vi "Lab Panel V5.22.vi"() -> ()   [LabVIEW 2013] (continued)
                    n2880 = Concatenate Strings("]", "\r") -> (w5216:string)
                    n2881 = Concatenate Strings(w5211, w5236, w5216) -> (w5226:string)
                    n2882 = Concatenate Strings(w5213, w5238, w5216) -> (w5228:string)
                    n2883 = Concatenate Strings(w5212, w5237, w5216) -> (w5227:string)
                    n2884 = Concatenate Strings(w5208, w5233, w5216) -> (w5223:string)
                    n2885 = Concatenate Strings(w5209, w5232, w5216) -> (w5224:string)
                    n2886 = Concatenate Strings(w5207, w5234, w5216) -> (w5222:string)
                    n2887 = Concatenate Strings(w5206, w5235, w5216) -> (w5221:string)
                    n2888 = Concatenate Strings(w5210, w5231, w5216) -> (w5225:string)
                    n2889 = Concatenate Strings(w5214, w5239, w5216) -> (w5229:string)
                    n2890 = Concatenate Strings(w5215, w5240, w5216) -> (w5230:string)
                    n2891 = Concatenate Strings(w5230, w5229, w5228, w5227, w5226, w5221, w5222, w5223, w5224, w5225) -> (w5199:string)
                    n2892 = Concatenate Strings("[PANEL/", "DESC/", "CYCLES/", "MINS/", "STATUS]", "\r", w5199) -> (w5198:string)
                    "MAIL REPORT" <- w5198
                    n2893 = global write "Global display 3.vi" "log all"(w5198) -> ()
                  }
                  frame #2 {
                    w5329 = "END"
                    n2894 = local read "mail control"() -> (w5330:string)
                    n2895 = case shown="False" w5325 {
                      tunnel: w5330 -> [w5354 _]
                      tunnel: w5329 -> [w5353 _]
                      tunnel: [w5352 FALSE] -> w5315
                      frame False {
                        n2896 = Equal?(x=w5354, y=w5353) -> (x = y?=w5352:bool)
                      }
                      frame True {
                      }
                    }
                    n2897 = case shown="False" w5331 {
                      tunnel: w5330 -> [w5370 _]
                      tunnel: w5329 -> [w5369 _]
                      tunnel: [w5368 FALSE] -> w5319
                      frame False {
                        n2898 = Equal?(x=w5370, y=w5369) -> (x = y?=w5368:bool)
                      }
                      frame True {
                      }
                    }
                    n2899 = case shown="False" w5328 {
                      tunnel: w5330 -> [w5366 _]
                      tunnel: w5329 -> [w5365 _]
                      tunnel: [w5364 FALSE] -> w5318
                      frame False {
                        n2900 = Equal?(x=w5366, y=w5365) -> (x = y?=w5364:bool)
                      }
                      frame True {
                      }
                    }
                    n2901 = case shown="False" w5326 {
                      tunnel: w5330 -> [w5358 _]
                      tunnel: w5329 -> [w5357 _]
                      tunnel: [w5356 FALSE] -> w5316
                      frame False {
                        n2902 = Equal?(x=w5358, y=w5357) -> (x = y?=w5356:bool)
                      }
                      frame True {
                      }
                    }
                    n2903 = case shown="False" w5327 {
                      tunnel: w5330 -> [w5362 _]
                      tunnel: w5329 -> [w5361 _]
                      tunnel: [w5360 FALSE] -> w5317
                      frame False {
                        n2904 = Equal?(x=w5362, y=w5361) -> (x = y?=w5360:bool)
                      }
                      frame True {
                      }
                    }
                    n2905 = Or(x=w5317, y=w5316) -> (x .or. y?=w5308:bool)
                    n2906 = Or(x=w5319, y=w5318) -> (x .or. y?=w5309:bool)
                    n2907 = Or(x=w5309, y=w5308) -> (x .or. y?=w5304:bool)
                    n2908 = case shown="False" w5321 {
                      tunnel: w5330 -> [w5338 _]
                      tunnel: w5329 -> [w5337 _]
                      tunnel: [w5336 FALSE] -> w5310
                      frame False {
                        n2909 = Equal?(x=w5338, y=w5337) -> (x = y?=w5336:bool)
                      }
                      frame True {
                      }
                    }
                    n2910 = case shown="False" w5320 {
                      tunnel: w5330 -> [w5334 _]
                      tunnel: w5329 -> [w5333 _]
                      tunnel: [w5332 FALSE] -> w5314
                      frame False {
                        n2911 = Equal?(x=w5334, y=w5333) -> (x = y?=w5332:bool)
                      }
                      frame True {
                      }
                    }
                    n2912 = case shown="False" w5322 {
                      tunnel: w5330 -> [w5342 _]
                      tunnel: w5329 -> [w5341 _]
                      tunnel: [w5340 FALSE] -> w5311
                      frame False {
                        n2913 = Equal?(x=w5342, y=w5341) -> (x = y?=w5340:bool)
                      }
                      frame True {
                      }
                    }
                    n2914 = case shown="False" w5324 {
                      tunnel: w5330 -> [w5350 _]
                      tunnel: w5329 -> [w5349 _]
                      tunnel: [w5348 FALSE] -> w5313
                      frame False {
                        n2915 = Equal?(x=w5350, y=w5349) -> (x = y?=w5348:bool)
                      }
                      frame True {
                      }
                    }
                    n2916 = case shown="False" w5323 {
                      tunnel: w5330 -> [w5346 _]
                      tunnel: w5329 -> [w5345 _]
                      tunnel: [w5344 FALSE] -> w5312
                      frame False {
                        n2917 = Equal?(x=w5346, y=w5345) -> (x = y?=w5344:bool)
                      }
                      frame True {
                      }
                    }
                    n2918 = Or(x=w5313, y=w5312) -> (x .or. y?=w5307:bool)
                    n2919 = Or(x=w5311, y=w5310) -> (x .or. y?=w5306:bool)
                    n2920 = Or(x=w5314, y=w5315) -> (x .or. y?=w5302:bool)
                    n2921 = Or(x=w5307, y=w5306) -> (x .or. y?=w5305:bool)
                    n2922 = Or(x=w5304, y=w5305) -> (x .or. y?=w5303:bool)
                    n2923 = Or(x=w5303, y=w5302) -> (x .or. y?=w5301:bool)
                  }
                  frame #3 {
                    n2924 = local read "on loops"() -> (w5384:dbl)
                    n2925 = local read "jig cycle"() -> (w5381:dbl)
                    n2926 = local read "Send Mail Now"() -> (w5375:bool)
                    n2927 = Add(x=w5384, y=3.0) -> (x+y=w5382:dbl)
                    n2928 = Equal?(x=w5381, y=w5382) -> (x = y?=w5376:bool)
                    n2929 = And(x=w5376, y=w5375) -> (x .and. y?=w5374:bool)
                    n2930 = And(x=w5380, y=w5376) -> (x .and. y?=w5379:bool)
                    n2931 = And(x=w5379, y=w5378) -> (x .and. y?=w5377:bool)
                    n2932 = Or(x=w5377, y=w5374) -> (x .or. y?=w5373:bool)
                    n2933 = case shown="True" w5373 {
                      tunnel: w5389 -> [_ w5395]
                      tunnel: w5388 -> [_ w5394]
                      tunnel: "Lab Panel Test Status" -> [_ w5393]
                      tunnel: w5386 -> [_ w5392]
                      tunnel: w5385 -> [_ w5391]
                      tunnel: w5372 -> [_ w5390]
                      frame False {
                      }
                      frame True {
                        n2934 = stacked-sequence {
                          tunnel: w5395 -> [w5403 _]
                          tunnel: w5394 -> [w5402 _]
                          tunnel: w5393 -> [w5401 _]
                          tunnel: w5392 -> [w5400 _]
                          tunnel: w5391 -> [w5399 _]
                          tunnel: w5390 -> [w5398 _]
                          frame #0 {
                            n2935 = call "sub vi - send mail v5.vi"("TO:"=w5403, "subject"=w5401, "from"=w5399, "out going server"=w5400, "message"=w5402) -> ("error out"=w5397:errorcluster)  [unwired: 10 in]
                            n2936 = Bundle(cluster=w5398, "mail error"=w5397) -> (w5396:T7)  [unwired: 6 in]
                            n2937 = local write "MAIL SETTINGS"(w5396) -> ()
                          }
                          frame #1 {
                            n2938 = local write "mail control"("") -> ()
                            n2939 = local write "Send Mail Now"(FALSE) -> ()
                          }
                        }
                      }
                    }
                  }
                }
              }
            }
          }
          frame #18 {
            # "save jig cycle values once all run switches are off"
            n2940 = stacked-sequence {
              tunnel: w5415 -> [_ w5444]
              tunnel: w5414 -> [_ w5443]
              tunnel: w5413 -> [_ w5442]
              tunnel: w5412 -> [_ w5441]
              tunnel: w5411 -> [_ w5440]
              tunnel: w5410 -> [_ w5439]
              tunnel: w5409 -> [_ w5438]
              tunnel: w5408 -> [_ w5437]
              tunnel: w5407 -> [_ w5436]
              tunnel: w5406 -> [_ w5435]
              frame #0 {
              }
              frame #1 {
                n2941 = Not(x=w5435) -> (.not. x?=w5418:bool)
                n2942 = Not(x=w5443) -> (.not. x?=w5433:bool)
                n2943 = Not(x=w5440) -> (.not. x?=w5428:bool)
                n2944 = Not(x=w5438) -> (.not. x?=w5424:bool)
                n2945 = Not(x=w5436) -> (.not. x?=w5420:bool)
                n2946 = Not(x=w5444) -> (.not. x?=w5434:bool)
                n2947 = Not(x=w5442) -> (.not. x?=w5432:bool)
                n2948 = Not(x=w5439) -> (.not. x?=w5426:bool)
                n2949 = Not(x=w5441) -> (.not. x?=w5430:bool)
                n2950 = Not(x=w5437) -> (.not. x?=w5422:bool)
                n2951 = local read "Save JC"() -> (w5446:bool)
                n2952 = And(x=w5434, y=w5433) -> (x .and. y?=w5431:bool)
                n2953 = And(x=w5431, y=w5432) -> (x .and. y?=w5429:bool)
                n2954 = And(x=w5429, y=w5430) -> (x .and. y?=w5427:bool)
                n2955 = And(x=w5427, y=w5428) -> (x .and. y?=w5425:bool)
                n2956 = And(x=w5425, y=w5426) -> (x .and. y?=w5423:bool)
                n2957 = And(x=w5423, y=w5424) -> (x .and. y?=w5421:bool)
                n2958 = And(x=w5421, y=w5422) -> (x .and. y?=w5419:bool)
                n2959 = And(x=w5419, y=w5420) -> (x .and. y?=w5417:bool)
                n2960 = And(x=w5417, y=w5418) -> (x .and. y?=w5416:bool)
                n2961 = And(x=w5416, y=w5446) -> (x .and. y?=w5445:bool)
                n2962 = case shown="True" w5445 {
                  tunnel: w5416 -> [w5447 _]
                  frame False {
                    n2963 = case shown="False" w5447 {
                      frame False {
                        n2964 = local write "Save JC"(TRUE) -> ()
                      }
                      frame True {
                      }
                    }
                  }
                  frame True {
                    n2965 = stacked-sequence {
                      frame #0 {
                        n2966 = String To Path(string="c:\\crabtree\\Jig Cycles\\") -> (path=w5459:path)
                        n2967 = Build Path(base path=w5459, name or relative path="jigcycles.bin") -> (appended path=w5457:path)
                        n2968 = Create Folder(path (use dialog)=w5459) -> (error out=w5461:errorcluster)  [unwired: 2 in, 2 out]
                        n2969 = local read "JIG RELAY CYCLES"() -> (w5451:T8)
                        n2970 = call <vilib>:"Clear Errors.vi"("error in (no error)"=w5461) -> ()  [unwired: 6 in, 1 out]
                        n2971 = local write "Save JC"(FALSE) -> ()
                        n2972 = Open/Create/Replace File(file path (use dialog)=w5457, operation (0:open)=T21."replace or create") -> (refnum out=w5455:refnum<file>, error out=w5456:errorcluster)  [unwired: 4 in, 1 out]
                        n2973 = Write to Binary File(file (use dialog)=w5455, data=w5451, error in=w5456) -> (refnum out=w5454:refnum<file>, error out=w5453:errorcluster)  [unwired: 3 in, 1 out]
                        n2974 = Close File(refnum=w5454, error in=w5453) -> (error out=w5452:errorcluster)  [unwired: 1 out]
                        n2975 = local write "data file error"(w5452) -> ()
                      }
                      frame #1 {
                        n2976 = local read "JIG RELAY CYCLES"() -> (w5484:T8)
                        n2977 = Unbundle By Name(w5484) -> ("LAB01-1"=w5479:dbl, "LAB01-2"=w5478:dbl, "LAB02-1"=w5476:dbl, "LAB02-2"=w5475:dbl, "LAB03-1"=w5473:dbl, "LAB03-2"=w5470:dbl, "LAB04-1"=w5469:dbl, "LAB04-2"=w5467:dbl, "LAB05-1"=w5465:dbl, "LAB05-2"=w5463:dbl)
                        n2978 = stacked-sequence {
                          tunnel: w5479 -> [w5487 _ _ _ _ _ _ _ _ _]
                          tunnel: 1000000 -> [w5490 w5500 w5510 w5520 w5530 w5540 w5550 w5560 w5570 w5580]
                          tunnel: [w5488 _ _ _ _ _ _ _ _ _] -> w5482
                          tunnel: "TEST STATION HAS REACHED 1 MILLION CYCLES, REPLACE  CONTROL RELAYS" -> [w5486 w5498 w5508 w5518 w5528 w5538 w5548 w5558 w5568 w5578]
                          tunnel: [_ w5497 _ _ _ _ _ _ _ _] -> w5480
                          tunnel: w5478 -> [_ w5496 _ _ _ _ _ _ _ _]
                          tunnel: [_ _ w5507 _ _ _ _ _ _ _] -> w5477
                          tunnel: w5476 -> [_ _ w5506 _ _ _ _ _ _ _]
                          tunnel: w5475 -> [_ _ _ w5517 _ _ _ _ _ _]
                          tunnel: [_ _ _ w5516 _ _ _ _ _ _] -> w5474
                          tunnel: w5473 -> [_ _ _ _ w5527 _ _ _ _ _]
                          tunnel: [_ _ _ _ w5526 _ _ _ _ _] -> w5472
                          tunnel: [_ _ _ _ _ w5537 _ _ _ _] -> w5471
                          tunnel: w5470 -> [_ _ _ _ _ w5536 _ _ _ _]
                          tunnel: w5469 -> [_ _ _ _ _ _ w5547 _ _ _]
                          tunnel: [_ _ _ _ _ _ w5546 _ _ _] -> w5468
                          tunnel: w5467 -> [_ _ _ _ _ _ _ w5557 _ _]
                          tunnel: [_ _ _ _ _ _ _ w5556 _ _] -> w5466
                          tunnel: w5465 -> [_ _ _ _ _ _ _ _ w5567 _]
                          tunnel: [_ _ _ _ _ _ _ _ w5566 _] -> w5464
                          tunnel: w5463 -> [_ _ _ _ _ _ _ _ _ w5577]
                          tunnel: [_ _ _ _ _ _ _ _ _ w5576] -> w5462
                          frame #0 {
                            n2979 = Greater?(x=w5487, y=w5490) -> (0:w5489:bool)
                            n2980 = case shown="True" w5489 {
                              tunnel: [w5491 0] -> w5488
                              tunnel: w5487 -> [w5491 _]
                              tunnel: w5486 -> [_ w5492]
                              frame False {
                              }
                              frame True {
                                n2981 = Concatenate Strings("LA01-1 ", w5492) -> (w5495:string)
                                n2982 = One Button Dialog(message=w5495) -> ()  [unwired: 1 in, 1 out]
                              }
                            }
                          }
                          frame #1 {
                            n2983 = Greater?(x=w5496, y=w5500) -> (0:w5499:bool)
                            n2984 = case shown="True" w5499 {
                              tunnel: [w5501 0] -> w5497
                              tunnel: w5496 -> [w5501 _]
                              tunnel: w5498 -> [_ w5502]
                              frame False {
                              }
                              frame True {
                                n2985 = Concatenate Strings("LA01-2 ", w5502) -> (w5505:string)
                                n2986 = One Button Dialog(message=w5505) -> ()  [unwired: 1 in, 1 out]
                              }
                            }
                          }
                          frame #2 {
                            n2987 = Greater?(x=w5506, y=w5510) -> (0:w5509:bool)
                            n2988 = case shown="True" w5509 {
                              tunnel: [w5511 0] -> w5507
                              tunnel: w5506 -> [w5511 _]
                              tunnel: w5508 -> [_ w5512]
                              frame False {
                              }
                              frame True {
                                n2989 = Concatenate Strings("LA02-1 ", w5512) -> (w5515:string)
                                n2990 = One Button Dialog(message=w5515) -> ()  [unwired: 1 in, 1 out]
                              }
                            }
                          }
                          frame #3 {
                            n2991 = Greater?(x=w5517, y=w5520) -> (0:w5519:bool)
                            n2992 = case shown="True" w5519 {
                              tunnel: [w5521 0] -> w5516
                              tunnel: w5517 -> [w5521 _]
                              tunnel: w5518 -> [_ w5522]
                              frame False {
                              }
                              frame True {
                                n2993 = Concatenate Strings("LA02-2 ", w5522) -> (w5525:string)
                                n2994 = One Button Dialog(message=w5525) -> ()  [unwired: 1 in, 1 out]
                              }
                            }
                          }
                          frame #4 {
                            n2995 = Greater?(x=w5527, y=w5530) -> (0:w5529:bool)
                            n2996 = case shown="True" w5529 {
                              tunnel: [w5531 0] -> w5526
                              tunnel: w5527 -> [w5531 _]
                              tunnel: w5528 -> [_ w5532]
                              frame False {
                              }
                              frame True {
                                n2997 = Concatenate Strings("LA03-1 ", w5532) -> (w5535:string)
                                n2998 = One Button Dialog(message=w5535) -> ()  [unwired: 1 in, 1 out]
                              }
                            }
                          }
                          frame #5 {
                            n2999 = Greater?(x=w5536, y=w5540) -> (0:w5539:bool)
                            n3000 = case shown="True" w5539 {
                              tunnel: [w5541 0] -> w5537
                              tunnel: w5536 -> [w5541 _]
                              tunnel: w5538 -> [_ w5542]
                              frame False {
                              }
                              frame True {
                                n3001 = Concatenate Strings("LA03-2 ", w5542) -> (w5545:string)
                                n3002 = One Button Dialog(message=w5545) -> ()  [unwired: 1 in, 1 out]
                              }
                            }
                          }
                          frame #6 {
                            n3003 = Greater?(x=w5547, y=w5550) -> (0:w5549:bool)
                            n3004 = case shown="True" w5549 {
                              tunnel: [w5551 0] -> w5546
                              tunnel: w5547 -> [w5551 _]
                              tunnel: w5548 -> [_ w5552]
                              frame False {
                              }
                              frame True {
                                n3005 = Concatenate Strings("LA04-1 ", w5552) -> (w5555:string)
                                n3006 = One Button Dialog(message=w5555) -> ()  [unwired: 1 in, 1 out]
                              }
                            }
                          }
                          frame #7 {
                            n3007 = Greater?(x=w5557, y=w5560) -> (0:w5559:bool)
                            n3008 = case shown="True" w5559 {
                              tunnel: [w5561 0] -> w5556
                              tunnel: w5557 -> [w5561 _]
                              tunnel: w5558 -> [_ w5562]
                              frame False {
                              }
                              frame True {
                                n3009 = Concatenate Strings("LA04-2 ", w5562) -> (w5565:string)
                                n3010 = One Button Dialog(message=w5565) -> ()  [unwired: 1 in, 1 out]
                              }
                            }
                          }
                          frame #8 {
                            n3011 = Greater?(x=w5567, y=w5570) -> (0:w5569:bool)
                            n3012 = case shown="True" w5569 {
                              tunnel: [w5571 0] -> w5566
                              tunnel: w5567 -> [w5571 _]
                              tunnel: w5568 -> [_ w5572]
                              frame False {
                              }
                              frame True {
                                n3013 = Concatenate Strings("LA05-1 ", w5572) -> (w5575:string)
                                n3014 = One Button Dialog(message=w5575) -> ()  [unwired: 1 in, 1 out]
                              }
                            }
                          }
                          frame #9 {
                            n3015 = Greater?(x=w5577, y=w5580) -> (0:w5579:bool)
                            n3016 = case shown="True" w5579 {
                              tunnel: [w5581 0] -> w5576
                              tunnel: w5577 -> [w5581 _]
                              tunnel: w5578 -> [_ w5582]
                              frame False {
                              }
                              frame True {
                                n3017 = Concatenate Strings("LA05-2 ", w5582) -> (w5585:string)
                                n3018 = One Button Dialog(message=w5585) -> ()  [unwired: 1 in, 1 out]
                              }
                            }
                          }
                        }
                        n3019 = Bundle By Name(cluster=w5484, "LAB01-1"=w5482, "LAB01-2"=w5480, "LAB02-1"=w5477, "LAB02-2"=w5474, "LAB03-1"=w5472, "LAB03-2"=w5471, "LAB04-1"=w5468, "LAB04-2"=w5466, "LAB05-1"=w5464, "LAB05-2"=w5462) -> (w5483:T8)
                        n3020 = local write "JIG RELAY CYCLES"(w5483) -> ()
                      }
                    }
                  }
                }
              }
            }
          }
          frame #19 {
            # "get temperature values"
            n3021 = local read "Panel #"() -> (w5586:dbl)
            n3022 = local read "Simulate"() -> (w5599:bool)
            n3023 = local read "Temp Test Cal"() -> (w5596:dbl)
            n3024 = stacked-sequence {
              seq-local: [w5602 _] -> [_ w5645]
              tunnel: w5599 -> [_ w5659]
              tunnel: T14 {"1  (A) cal"=1.0, "1 (V) cal"=1.0, "1 (PF) cal"=1.0, "1 (TL) cal"=1.0, "1 (TN) cal"=1.0, "2 (A) cal"=1.0, "2 (V) cal"=1.0, "2 (PF) cal"=1.0, "2 (TL) cal"=1.0, "2 (TN) cal"=1.0} ("CAL LAB01") -> [_ w5658]
              tunnel: w5597 -> [_ w5657]
              tunnel: w5596 -> [_ w5656]
              tunnel: w5595 -> [_ w5655]
              tunnel: w5594 -> [_ w5654]
              tunnel: w5593 -> [_ w5653]
              tunnel: w5592 -> [_ w5652]
              tunnel: w5591 -> [_ w5651]
              tunnel: w5590 -> [_ w5650]
              tunnel: w5589 -> [_ w5649]
              tunnel: w5588 -> [_ w5648]
              tunnel: w5587 -> [_ w5647]
              tunnel: w5586 -> [_ w5646]
              frame #0 {
                n3025 = local read "Select COM port"() -> (w5603:refnum<visa-resource-name>)
                "COM port" <- w5603
                n3026 = global write "Global 1.vi" "COM port"(w5603) -> ()
                n3027 = global write "Global 1.vi" "tmp dly lps"("Temp Delay Lps") -> ()
                n3028 = global write "Global 1.vi" "dly value"("Temp Value") -> ()
                n3029 = local read "jig cycle"() -> (w5605:dbl)
                n3030 = local read "on loops"() -> (w5607:dbl)
                n3031 = Add(x=w5607, y=3) -> (x+y=w5608:dbl)
                n3032 = local read "Panel #"() -> (w5604:dbl)
                n3033 = Equal?(x=w5605, y=w5608) -> (x = y?=w5602:bool)
                n3034 = case shown="True" w5602 {
                  tunnel: w5604 -> [_ w5613]
                  frame False {
                  }
                  frame True {
                    n3035 = local read "Simulate"() -> (w5610:bool)
                    n3036 = case shown="1" w5613 {
                      tunnel: 1.0 -> [_ w5620 w5623 w5630 w5635 w5641]
                      tunnel: w5610 -> [_ w5616 w5622 w5628 w5636 w5640]
                      tunnel: [FALSE w5615 w5621 w5627 w5633 w5639] -> w5609
                      frame 0, Default {
                      }
                      frame 1 {
                        w5618 = FALSE
                        n3037 = call "sub vi - GET ALL TEMP v7.vi"("LA01-EN"=TRUE, "simulate"=w5616, "LA02-EN"=w5618, "LA03-EN"=w5618, "LA04-EN"=w5618, "LA05-EN"=w5618, "Gen Cal Value"=w5620) -> ("LA01 TEMP"=w5617:T24, "error"=w5615:bool)  [unwired: 3 in, 4 out]
                        n3038 = local write "LAB01 TEMP"(w5617) -> ()
                      }
                      frame 2 {
                        w5624 = FALSE
                        n3039 = call "sub vi - GET ALL TEMP v7.vi"("LA01-EN"=w5624, "simulate"=w5622, "LA02-EN"=TRUE, "LA03-EN"=w5624, "LA04-EN"=w5624, "LA05-EN"=w5624, "Gen Cal Value"=w5623) -> ("LA02 TEMP"=w5626:T24, "error"=w5621:bool)  [unwired: 3 in, 4 out]
                        n3040 = local write "LAB02 TEMP"(w5626) -> ()
                      }
                      frame 3 {
                        w5631 = FALSE
                        n3041 = call "sub vi - GET ALL TEMP v7.vi"("LA01-EN"=w5631, "simulate"=w5628, "LA02-EN"=w5631, "LA03-EN"=TRUE, "LA04-EN"=w5631, "LA05-EN"=w5631, "Gen Cal Value"=w5630) -> ("LA03 TEMP"=w5629:T24, "error"=w5627:bool)  [unwired: 3 in, 4 out]
                        n3042 = local write "LAB03 TEMP"(w5629) -> ()
                      }
                      frame 4 {
                        w5637 = FALSE
                        n3043 = call "sub vi - GET ALL TEMP v7.vi"("LA01-EN"=w5637, "simulate"=w5636, "LA02-EN"=w5637, "LA03-EN"=w5637, "LA04-EN"=TRUE, "LA05-EN"=w5637, "Gen Cal Value"=w5635) -> ("LA04 TEMP"=w5634:T24, "error"=w5633:bool)  [unwired: 3 in, 4 out]
                        n3044 = local write "LAB04 TEMP"(w5634) -> ()
                      }
                      frame 5 {
                        w5643 = FALSE
                        n3045 = call "sub vi - GET ALL TEMP v7.vi"("LA01-EN"=w5643, "simulate"=w5640, "LA02-EN"=w5643, "LA03-EN"=w5643, "LA04-EN"=w5643, "LA05-EN"=TRUE, "Gen Cal Value"=w5641) -> ("error"=w5639:bool, "LA05 TEMP"=w5642:T24)  [unwired: 3 in, 4 out]
                        n3046 = local write "LAB05 TEMP"(w5642) -> ()
                      }
                    }
                    "Error Temp" <- w5609
                    n3047 = local write "TEMP"(TRUE) -> ()
                  }
                }
              }
              frame #1 {
                n3048 = case shown="True" w5645 {
                  tunnel: w5659 -> [_ w5673]
                  tunnel: w5658 -> [_ w5672]
                  tunnel: w5657 -> [_ w5671]
                  tunnel: w5656 -> [_ w5670]
                  tunnel: w5655 -> [_ w5669]
                  tunnel: w5654 -> [_ w5668]
                  tunnel: w5653 -> [_ w5667]
                  tunnel: w5652 -> [_ w5666]
                  tunnel: w5651 -> [_ w5665]
                  tunnel: w5650 -> [_ w5664]
                  tunnel: w5649 -> [_ w5663]
                  tunnel: w5648 -> [_ w5662]
                  tunnel: w5647 -> [_ w5661]
                  tunnel: w5646 -> [_ w5660]
                  frame False {
                  }
                  frame True {
                    n3049 = case shown="1" w5660 {
                      tunnel: w5673 -> [_ w5686 w5731 w5776 w5821 w5866]
                      tunnel: w5672 -> [_ w5685 w5730 w5775 w5820 w5865]
                      tunnel: w5671 -> [_ w5675 _ _ _ _]
                      tunnel: w5670 -> [_ w5680 w5729 w5774 w5819 w5864]
                      tunnel: w5669 -> [_ w5674 _ _ _ _]
                      tunnel: w5668 -> [_ _ w5720 _ _ _]
                      tunnel: w5667 -> [_ _ w5719 _ _ _]
                      tunnel: w5666 -> [_ _ _ w5765 _ _]
                      tunnel: w5665 -> [_ _ _ w5764 _ _]
                      tunnel: w5664 -> [_ _ _ _ w5810 _]
                      tunnel: w5663 -> [_ _ _ _ w5809 _]
                      tunnel: w5662 -> [_ _ _ _ _ w5855]
                      tunnel: w5661 -> [_ _ _ _ _ w5854]
                      frame ..0 {
                      }
                      frame 1 {
                        n3050 = case shown="False" w5686 {
                          tunnel: [w5717 w5718] -> w5702
                          tunnel: w5685 -> [_ w5718]
                          frame False {
                            n3051 = local read "CAL LAB01"() -> (w5717:T14)
                          }
                          frame True {
                          }
                        }
                        n3052 = local read "TEMP LA01"() -> (w5693:T9)
                        n3053 = local read "LAB01 TEMP"() -> (w5692:T12)
                        n3054 = call "sub vi - temperature delay v3.vi"("2-run"=w5674, "1-run"=w5675, "temp values IN"=w5693, "temp signals"=w5692) -> ("T2-N"=w5688:dbl, "T2-L"=w5689:dbl, "T1-N"=w5690:dbl, "T1-L"=w5691:dbl, "temp values OUT"=w5687:T43)  [unwired: 3 in]
                        n3055 = Unbundle By Name(w5702) -> ("1 (TL) cal"=w5697:dbl, "1 (TN) cal"=w5696:dbl, "2 (TL) cal"=w5695:dbl, "2 (TN) cal"=w5694:dbl)  [unwired: 6 out]
                        n3056 = local write "TEMP LA01"(w5687) -> ()
                        n3057 = Multiply(x=w5691, y=w5697) -> (x*y=w5684:dbl)
                        n3058 = Multiply(x=w5690, y=w5696) -> (x*y=w5682:dbl)
                        n3059 = Multiply(x=w5689, y=w5695) -> (x*y=w5679:dbl)
                        n3060 = Multiply(x=w5688, y=w5694) -> (x*y=w5678:dbl)
                        n3061 = case shown="True" w5675 {
                          tunnel: w5684 -> [w5711 w5716]
                          tunnel: w5680 -> [_ w5714]
                          tunnel: [w5711 w5715] -> w5683
                          tunnel: w5682 -> [w5710 w5713]
                          tunnel: [w5710 w5712] -> w5681
                          frame False {
                          }
                          frame True {
                            n3062 = Multiply(x=w5714, y=w5713) -> (x*y=w5712:dbl)
                            n3063 = Multiply(x=w5714, y=w5716) -> (x*y=w5715:dbl)
                          }
                        }
                        n3064 = case shown="True" w5674 {
                          tunnel: w5679 -> [w5704 w5709]
                          tunnel: w5680 -> [_ w5707]
                          tunnel: [w5704 w5708] -> w5677
                          tunnel: w5678 -> [w5703 w5706]
                          tunnel: [w5703 w5705] -> w5676
                          frame False {
                          }
                          frame True {
                            n3065 = Multiply(x=w5707, y=w5706) -> (x*y=w5705:dbl)
                            n3066 = Multiply(x=w5707, y=w5709) -> (x*y=w5708:dbl)
                          }
                        }
                        n3067 = local read "SIG LAB01-2"() -> (w5699:T2)
                        n3068 = local read "SIG LAB01-1"() -> (w5701:T2)
                        n3069 = Bundle By Name(cluster=w5701, "Tmp Live"=w5683, "Tmp Neut"=w5681) -> (w5700:T2)
                        n3070 = Bundle By Name(cluster=w5699, "Tmp Live"=w5677, "Tmp Neut"=w5676) -> (w5698:T2)
                        n3071 = local write "SIG LAB01-1"(w5700) -> ()
                        n3072 = local write "SIG LAB01-2"(w5698) -> ()
                      }
                      frame 2 {
                        n3073 = case shown="True" w5731 {
                          tunnel: [w5762 w5763] -> w5747
                          tunnel: w5730 -> [_ w5763]
                          frame False {
                            n3074 = local read "CAL LAB02"() -> (w5762:T15)
                          }
                          frame True {
                          }
                        }
                        n3075 = local read "LAB02 TEMP"() -> (w5738:T12)
                        n3076 = local read "TEMP LA02"() -> (w5737:T9)
                        n3077 = call "sub vi - temperature delay v3.vi"("2-run"=w5719, "1-run"=w5720, "temp values IN"=w5737, "temp signals"=w5738) -> ("T2-N"=w5732:dbl, "T2-L"=w5733:dbl, "T1-N"=w5734:dbl, "T1-L"=w5735:dbl, "temp values OUT"=w5736:T43)  [unwired: 3 in]
                        n3078 = Unbundle By Name(w5747) -> ("1 (TL) cal"=w5742:dbl, "1 (TN) cal"=w5741:dbl, "2 (TL) cal"=w5740:dbl, "2 (TN) cal"=w5739:dbl)  [unwired: 6 out]
                        n3079 = local write "TEMP LA02"(w5736) -> ()
                        n3080 = Multiply(x=w5735, y=w5742) -> (x*y=w5728:dbl)
                        n3081 = Multiply(x=w5734, y=w5741) -> (x*y=w5727:dbl)
                        n3082 = Multiply(x=w5733, y=w5740) -> (x*y=w5724:dbl)
                        n3083 = Multiply(x=w5732, y=w5739) -> (x*y=w5723:dbl)
                        n3084 = case shown="True" w5720 {
                          tunnel: w5728 -> [w5756 w5761]
                          tunnel: w5729 -> [_ w5759]
                          tunnel: [w5756 w5760] -> w5726
                          tunnel: w5727 -> [w5755 w5758]
                          tunnel: [w5755 w5757] -> w5725
                          frame False {
                          }
                          frame True {
                            n3085 = Multiply(x=w5759, y=w5758) -> (x*y=w5757:dbl)
                            n3086 = Multiply(x=w5759, y=w5761) -> (x*y=w5760:dbl)
                          }
                        }
                        n3087 = case shown="True" w5719 {
                          tunnel: w5724 -> [w5749 w5754]
                          tunnel: w5729 -> [_ w5752]
                          tunnel: [w5749 w5753] -> w5722
                          tunnel: w5723 -> [w5748 w5751]
                          tunnel: [w5748 w5750] -> w5721
                          frame False {
                          }
                          frame True {
                            n3088 = Multiply(x=w5752, y=w5751) -> (x*y=w5750:dbl)
                            n3089 = Multiply(x=w5752, y=w5754) -> (x*y=w5753:dbl)
                          }
                        }
                        n3090 = local read "SIG LAB02-2"() -> (w5744:T2)
                        n3091 = local read "SIG LAB02-1"() -> (w5746:T2)
                        n3092 = Bundle By Name(cluster=w5746, "Tmp Live"=w5726, "Tmp Neut"=w5725) -> (w5745:T2)
                        n3093 = Bundle By Name(cluster=w5744, "Tmp Live"=w5722, "Tmp Neut"=w5721) -> (w5743:T2)
                        n3094 = local write "SIG LAB02-1"(w5745) -> ()
                        n3095 = local write "SIG LAB02-2"(w5743) -> ()
                      }
                      frame 3 {
                        n3096 = case shown="False" w5776 {
                          tunnel: [w5807 w5808] -> w5792
                          tunnel: w5775 -> [_ w5808]
                          frame False {
                            n3097 = local read "CAL LAB03"() -> (w5807:T14)
                          }
                          frame True {
                          }
                        }
                        n3098 = local read "TEMP LA03"() -> (w5782:T9)
                        n3099 = local read "LAB03 TEMP"() -> (w5783:T12)
                        n3100 = call "sub vi - temperature delay v3.vi"("2-run"=w5764, "1-run"=w5765, "temp values IN"=w5782, "temp signals"=w5783) -> ("T2-N"=w5777:dbl, "T2-L"=w5778:dbl, "T1-N"=w5779:dbl, "T1-L"=w5780:dbl, "temp values OUT"=w5781:T43)  [unwired: 3 in]
                        n3101 = Unbundle By Name(w5792) -> ("1 (TL) cal"=w5787:dbl, "1 (TN) cal"=w5786:dbl, "2 (TL) cal"=w5785:dbl, "2 (TN) cal"=w5784:dbl)  [unwired: 6 out]
                        n3102 = local write "TEMP LA03"(w5781) -> ()
                        n3103 = Multiply(x=w5780, y=w5787) -> (x*y=w5773:dbl)
                        n3104 = Multiply(x=w5779, y=w5786) -> (x*y=w5772:dbl)
                        n3105 = Multiply(x=w5778, y=w5785) -> (x*y=w5769:dbl)
                        n3106 = Multiply(x=w5777, y=w5784) -> (x*y=w5768:dbl)
                        n3107 = case shown="True" w5764 {
                          tunnel: w5769 -> [w5794 w5799]
                          tunnel: w5774 -> [_ w5797]
                          tunnel: [w5794 w5798] -> w5767
                          tunnel: w5768 -> [w5793 w5796]
                          tunnel: [w5793 w5795] -> w5766
                          frame False {
                          }
                          frame True {
                            n3108 = Multiply(x=w5797, y=w5796) -> (x*y=w5795:dbl)
                            n3109 = Multiply(x=w5797, y=w5799) -> (x*y=w5798:dbl)
                          }
                        }
                        n3110 = case shown="True" w5765 {
                          tunnel: w5773 -> [w5801 w5806]
                          tunnel: w5774 -> [_ w5804]
                          tunnel: [w5801 w5805] -> w5771
                          tunnel: w5772 -> [w5800 w5803]
                          tunnel: [w5800 w5802] -> w5770
                          frame False {
                          }
                          frame True {
                            n3111 = Multiply(x=w5804, y=w5803) -> (x*y=w5802:dbl)
                            n3112 = Multiply(x=w5804, y=w5806) -> (x*y=w5805:dbl)
                          }
                        }
                        n3113 = local read "SIG LAB03-2"() -> (w5789:T2)
                        n3114 = local read "SIG LAB03-1"() -> (w5791:T2)
                        n3115 = Bundle By Name(cluster=w5791, "Tmp Live"=w5771, "Tmp Neut"=w5770) -> (w5790:T2)
                        n3116 = Bundle By Name(cluster=w5789, "Tmp Live"=w5767, "Tmp Neut"=w5766) -> (w5788:T2)
                        n3117 = local write "SIG LAB03-1"(w5790) -> ()
                        n3118 = local write "SIG LAB03-2"(w5788) -> ()
                      }
                      frame 4 {
                        n3119 = case shown="False" w5821 {
                          tunnel: [w5852 w5853] -> w5837
                          tunnel: w5820 -> [_ w5853]
                          frame False {
                            n3120 = local read "CAL LAB04"() -> (w5852:T14)
                          }
                          frame True {
                          }
                        }
                        n3121 = local read "LAB04 TEMP"() -> (w5827:T12)
                        n3122 = local read "TEMP LA04"() -> (w5828:T9)
                        n3123 = call "sub vi - temperature delay v3.vi"("2-run"=w5809, "1-run"=w5810, "temp values IN"=w5828, "temp signals"=w5827) -> ("T2-N"=w5822:dbl, "T2-L"=w5823:dbl, "T1-N"=w5824:dbl, "T1-L"=w5825:dbl, "temp values OUT"=w5826:T43)  [unwired: 3 in]
                        n3124 = Unbundle By Name(w5837) -> ("1 (TL) cal"=w5832:dbl, "1 (TN) cal"=w5831:dbl, "2 (TL) cal"=w5830:dbl, "2 (TN) cal"=w5829:dbl)  [unwired: 6 out]
                        n3125 = local write "TEMP LA04"(w5826) -> ()
                        n3126 = Multiply(x=w5825, y=w5832) -> (x*y=w5818:dbl)
                        n3127 = Multiply(x=w5824, y=w5831) -> (x*y=w5817:dbl)
                        n3128 = Multiply(x=w5823, y=w5830) -> (x*y=w5814:dbl)
                        n3129 = Multiply(x=w5822, y=w5829) -> (x*y=w5813:dbl)
                        n3130 = case shown="True" w5809 {
                          tunnel: w5814 -> [w5839 w5844]
                          tunnel: w5819 -> [_ w5842]
                          tunnel: [w5839 w5843] -> w5812
                          tunnel: w5813 -> [w5838 w5841]
                          tunnel: [w5838 w5840] -> w5811
                          frame False {
                          }
                          frame True {
                            n3131 = Multiply(x=w5842, y=w5841) -> (x*y=w5840:dbl)
                            n3132 = Multiply(x=w5842, y=w5844) -> (x*y=w5843:dbl)
                          }
                        }
                        n3133 = case shown="True" w5810 {
                          tunnel: w5818 -> [w5846 w5851]
                          tunnel: w5819 -> [_ w5849]
                          tunnel: [w5846 w5850] -> w5816
                          tunnel: w5817 -> [w5845 w5848]
                          tunnel: [w5845 w5847] -> w5815
                          frame False {
                          }
                          frame True {
                            n3134 = Multiply(x=w5849, y=w5848) -> (x*y=w5847:dbl)
                            n3135 = Multiply(x=w5849, y=w5851) -> (x*y=w5850:dbl)
                          }
                        }
                        n3136 = local read "SIG LAB04-2"() -> (w5834:T2)
                        n3137 = local read "SIG LAB04-1"() -> (w5836:T2)
                        n3138 = Bundle By Name(cluster=w5836, "Tmp Live"=w5816, "Tmp Neut"=w5815) -> (w5835:T2)
                        n3139 = Bundle By Name(cluster=w5834, "Tmp Live"=w5812, "Tmp Neut"=w5811) -> (w5833:T2)
                        n3140 = local write "SIG LAB04-1"(w5835) -> ()
                        n3141 = local write "SIG LAB04-2"(w5833) -> ()
                      }
                      frame 5.. {
                        n3142 = case shown="False" w5866 {
                          tunnel: [w5897 w5898] -> w5882
                          tunnel: w5865 -> [_ w5898]
                          frame False {
                            n3143 = local read "CAL LAB05"() -> (w5897:T14)
                          }
                          frame True {
                          }
                        }
                        n3144 = local read "LAB05 TEMP"() -> (w5872:T12)
                        n3145 = local read "TEMP LA05"() -> (w5873:T9)
                        n3146 = call "sub vi - temperature delay v3.vi"("2-run"=w5854, "1-run"=w5855, "temp values IN"=w5873, "temp signals"=w5872) -> ("T2-N"=w5868:dbl, "T2-L"=w5869:dbl, "T1-N"=w5870:dbl, "T1-L"=w5871:dbl, "temp values OUT"=w5867:T43)  [unwired: 3 in]
                        n3147 = local write "TEMP LA05"(w5867) -> ()
                        n3148 = Unbundle By Name(w5882) -> ("1 (TL) cal"=w5874:dbl, "1 (TN) cal"=w5877:dbl, "2 (TL) cal"=w5876:dbl, "2 (TN) cal"=w5875:dbl)  [unwired: 6 out]
                        n3149 = Multiply(x=w5871, y=w5874) -> (x*y=w5863:dbl)
                        n3150 = Multiply(x=w5870, y=w5877) -> (x*y=w5862:dbl)
                        n3151 = Multiply(x=w5869, y=w5876) -> (x*y=w5859:dbl)
                        n3152 = Multiply(x=w5868, y=w5875) -> (x*y=w5858:dbl)
                        n3153 = case shown="True" w5854 {
                          tunnel: w5859 -> [w5884 w5889]
                          tunnel: w5864 -> [_ w5887]
                          tunnel: [w5884 w5888] -> w5857
                          tunnel: w5858 -> [w5883 w5886]
                          tunnel: [w5883 w5885] -> w5856
                          frame False {
                          }
                          frame True {
                            n3154 = Multiply(x=w5887, y=w5886) -> (x*y=w5885:dbl)
                            n3155 = Multiply(x=w5887, y=w5889) -> (x*y=w5888:dbl)
                          }
                        }
                        n3156 = case shown="True" w5855 {
                          tunnel: w5863 -> [w5891 w5896]
                          tunnel: w5864 -> [_ w5894]
                          tunnel: [w5891 w5895] -> w5861
                          tunnel: w5862 -> [w5890 w5893]
                          tunnel: [w5890 w5892] -> w5860
                          frame False {
                          }
                          frame True {
                            n3157 = Multiply(x=w5894, y=w5893) -> (x*y=w5892:dbl)
                            n3158 = Multiply(x=w5894, y=w5896) -> (x*y=w5895:dbl)
                          }
                        }
                        n3159 = local read "SIG LAB05-1"() -> (w5881:T2)
                        n3160 = Bundle By Name(cluster=w5881, "Tmp Live"=w5861, "Tmp Neut"=w5860) -> (w5880:T2)
                        n3161 = local read "SIG LAB05-2"() -> (w5879:T2)
                        n3162 = Bundle By Name(cluster=w5879, "Tmp Live"=w5857, "Tmp Neut"=w5856) -> (w5878:T2)
                        n3163 = local write "SIG LAB05-1"(w5880) -> ()
                        n3164 = local write "SIG LAB05-2"(w5878) -> ()
                      }
                    }
                  }
                }
              }
            }
          }
          frame #20 {
            # "write data to display panel"
            n3165 = global write "Global display 1.vi" "TEST 5-2"(w5933) -> ()
            n3166 = global write "Global display 1.vi" "TEST 4-2"(w5935) -> ()
            n3167 = global write "Global display 1.vi" "TEST 1-2"(w5941) -> ()
            n3168 = global write "Global display 1.vi" "TEST 3-1"(w5938) -> ()
            n3169 = global write "Global display 1.vi" "TEST 5-1"(w5934) -> ()
            n3170 = global write "Global display 1.vi" "TEST 1-1"(w5942) -> ()
            n3171 = global write "Global display 1.vi" "TEST 3-2"(w5937) -> ()
            n3172 = global write "Global display 1.vi" "TEST 4-1"(w5936) -> ()
            n3173 = global write "Global display 1.vi" "TEST 2-2"(w5939) -> ()
            n3174 = global write "Global display 1.vi" "TEST 2-1"(w5940) -> ()
            n3175 = global read "Global display 3.vi" "log 1-1"() -> (→"LOG LAB01-1":string)
            n3176 = global read "Global display 3.vi" "log 3-1"() -> (→"LOG LAB03-1":string)
            n3177 = global read "Global display 3.vi" "log 1-2"() -> (→"LOG LAB01-2":string)
            n3178 = property on="Tab Control 2" class="TabCtl (strict)"() -> ("Pages"=w5932:refnum<vi>[])  [unwired: 2 in, 2 out]
            n3179 = global read "Global display 3.vi" "log 2-1"() -> (→"LOG LAB02-1":string)
            n3180 = global read "Global display 3.vi" "log 2-2"() -> (→"LOG LAB02-2":string)
            n3181 = global read "Global display 3.vi" "log 4-2"() -> (→"LOG LAB04-2":string)
            n3182 = global read "Global display 3.vi" "log 5-2"() -> (→"LOG LAB05-2":string)
            n3183 = global read "Global display 3.vi" "log 5-1"() -> (→"LOG LAB05-1":string)
            n3184 = global read "Global display 3.vi" "log 4-1"() -> (→"LOG LAB04-1":string)
            n3185 = global read "Global display 3.vi" "log 3-2"() -> (→"LOG LAB03-2":string)
            n3186 = Index Array(array=w5932, index=8) -> (element=w5930:refnum<vi>)
            n3187 = property class="Page"(reference=w5930) -> ("PageVis"=w5929:bool)  [unwired: 1 in, 2 out]
            n3188 = global write "Global display 3.vi" "admin"(w5929) -> ()
            n3189 = local read "O/I  LAB05-2"() -> (w5983:bool)
            n3190 = local read "O/I  LAB05-1"() -> (w5984:bool)
            n3191 = local read "O/I  LAB03-2"() -> (w5987:bool)
            n3192 = local read "O/I  LAB04-2"() -> (w5985:bool)
            n3193 = local read "O/I  LAB04-1"() -> (w5986:bool)
            n3194 = local read "O/I  LAB03-1"() -> (w5988:bool)
            n3195 = local read "O/I  LAB01-2"() -> (w5991:bool)
            n3196 = local read "O/I  LAB01-1"() -> (w5992:bool)
            n3197 = local read "O/I  LAB02-1"() -> (w5990:bool)
            n3198 = local read "O/I  LAB02-2"() -> (w5989:bool)
            n3199 = global write "Global display 1.vi" "5-2 O/F"(w5983) -> ()
            n3200 = global write "Global display 1.vi" "5-1 O/F"(w5984) -> ()
            n3201 = global write "Global display 1.vi" "4-1 O/F"(w5986) -> ()
            n3202 = global write "Global display 1.vi" "4-2 O/F"(w5985) -> ()
            n3203 = global write "Global display 1.vi" "3-2 O/F"(w5987) -> ()
            n3204 = global write "Global display 1.vi" "3-1 O/F"(w5988) -> ()
            n3205 = global write "Global display 1.vi" "2-2 O/F"(w5989) -> ()
            n3206 = global write "Global display 1.vi" "2-1 O/F"(w5990) -> ()
            n3207 = global write "Global display 1.vi" "1-2 O/F"(w5991) -> ()
            n3208 = global write "Global display 1.vi" "1-1 O/F"(w5992) -> ()
            n3209 = local read "TEMP START LAB02-2"() -> (w5915:cluster{"TL":dbl, "TN":dbl})
            n3210 = local read "run lab05-2"() -> (w5973:bool)
            n3211 = local read "TEMP START LAB01-2"() -> (w5917:cluster{"TL":dbl, "TN":dbl})
            n3212 = local read "TEMP START LAB02-1"() -> (w5916:cluster{"TL":dbl, "TN":dbl})
            n3213 = local read "TEMP START LAB04-1"() -> (w5912:cluster{"TL":dbl, "TN":dbl})
            n3214 = local read "TEMP START LAB04-2"() -> (w5911:cluster{"TL":dbl, "TN":dbl})
            n3215 = local read "run lab04-1"() -> (w5976:bool)
            n3216 = local read "run lab04-2"() -> (w5975:bool)
            n3217 = local read "run lab05-1"() -> (w5974:bool)
